vi "ChangePanel.vi"(8 "error in (no error)":errorcluster, 9 "New Active Index":i32, 10 "Panel Index":i32, 11 "MAUI in":refnum<class "SMO.UI.MAUI.lvclass">) -> (0 "error out":errorcluster, 3 "MAUI out":refnum<class "SMO.UI.MAUI.lvclass">)   [LabVIEW 2020, in "SMO.UI.MAUI.lvclass"]
uses:
  SMO.UI.MAUI.lvclass
  SMO.UI.MAUI.lvclass/SMO.UI.MAUI.ctl
  <vilib>/Levylab/SMO.UI.Embedded/SMO.UI.Embedded.lvclass
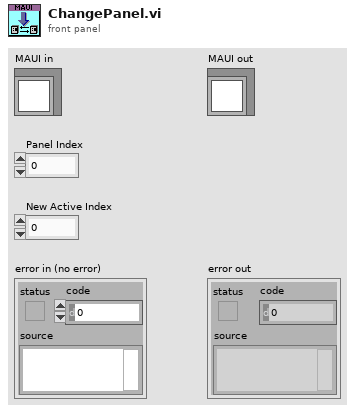
[diagram p1: front panel]
types:
  T1 = typedef "SMO.UI.MAUI.lvclass/PanelData.ctl" = cluster{"SubPanel":refnum<vi>, "Ring":refnum<vi>, "Active":i32}
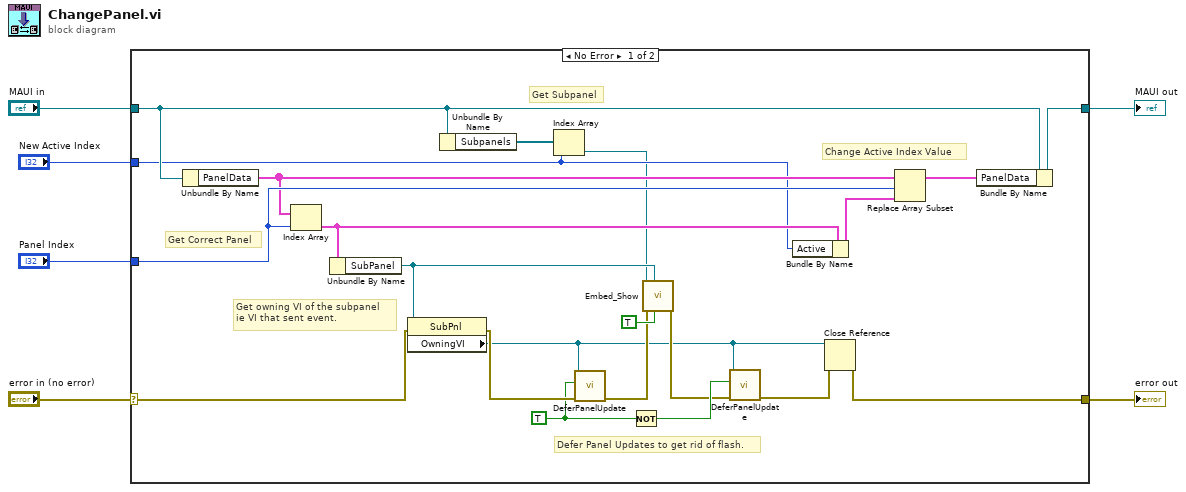
[diagram p0: block diagram]
diagram:
  n1 = case shown="No Error" "error in (no error)" {
    selector: "error in (no error)" -> [w21 w29]
    tunnel: [w17 w29] -> w5
    tunnel: [w22 w28] -> w3
    tunnel: "MAUI in" -> [w23 w28]
    tunnel: "Panel Index" -> [w24 _]
    tunnel: "New Active Index" -> [w18 _]
    frame No Error {
      w11 = TRUE
      # "Defer Panel Updates to get rid of flash."
      # "Get owning VI of the subpanel\nie VI that sent event."
      # "Get Subpanel"
      # "Change Active Index Value"
      # "Get Correct Panel"
      n2 = Unbundle By Name(w23) -> ("PanelData"=w20:T1[])
      n3 = Index Array(array=w20, index=w24) -> (element=w26:T1)
      n4 = Unbundle By Name(w26) -> ("SubPanel"=w16:refnum<vi>)
      n5 = property on="Property Node" class="SubPnl"(reference=w16, error in=w21) -> (error out=w13:errorcluster, "OwningVI"=w7:refnum<vi>)  [unwired: 1 out]
      n6 = Unbundle By Name(w23) -> ("Subpanels"=w27:refnum<class "SMO.UI.Embedded.lvclass">[])
      n7 = Index Array(array=w27, index=w18) -> (element=w15:refnum<class "SMO.UI.Embedded.lvclass">)
      n8 = call <vilib>:"DeferPanelUpdate.vi"("error in (no error)"=w13, "Defer Panel Updates"=w11, "VI in"=w7) -> ("error out"=w12:errorcluster)  [unwired: 8 in]
      n9 = Not(x=w11) -> (.not. x?=w10:bool)
      n10 = call <vilib>:"Embed_Show.vi"("Force?"=TRUE, "Sub Panel"=w16, "error in (no error)"=w12, "EmbeddedSMO in"=w15) -> ("error out"=w9:errorcluster)  [unwired: 6 in, 1 out]
      n11 = call <vilib>:"DeferPanelUpdate.vi"("error in (no error)"=w9, "Defer Panel Updates"=w10, "VI in"=w7) -> ("error out"=w8:errorcluster)  [unwired: 8 in]
      n12 = Bundle By Name(cluster=w26, "Active"=w18) -> (w25:T1)
      n13 = Close Reference(reference=w7, error in (no error)=w8) -> (error out=w17:errorcluster)
      n14 = Replace Array Subset(array=w20, new element=w25, index=w24) -> (w19:T1[])
      n15 = Bundle By Name(cluster=w23, "PanelData"=w19) -> (w22:refnum<class "SMO.UI.MAUI.lvclass">)
    }
    frame Error {
    }
  }
  "error out" <- w5
  "MAUI out" <- w3
